vi "FourierSeries.vi"() -> ()   [LabVIEW 2020]
uses:
  <vilib>/Analysis/2dsp.llb/Real FFT.vi
  <vilib>/measure/NI_MABase.lvlib
  <vilib>/Analysis/NI_AALPro.lvlib
panel:
  out "Square Wave 2":dbl[](graph)
  out "FFT {X}":cdb[](array[numeric])
  out "Square Wave":waveform(dbl)(graph)
  in  "Frequency 2":dbl
  in  "Frequency":dbl
  in  "K":dbl
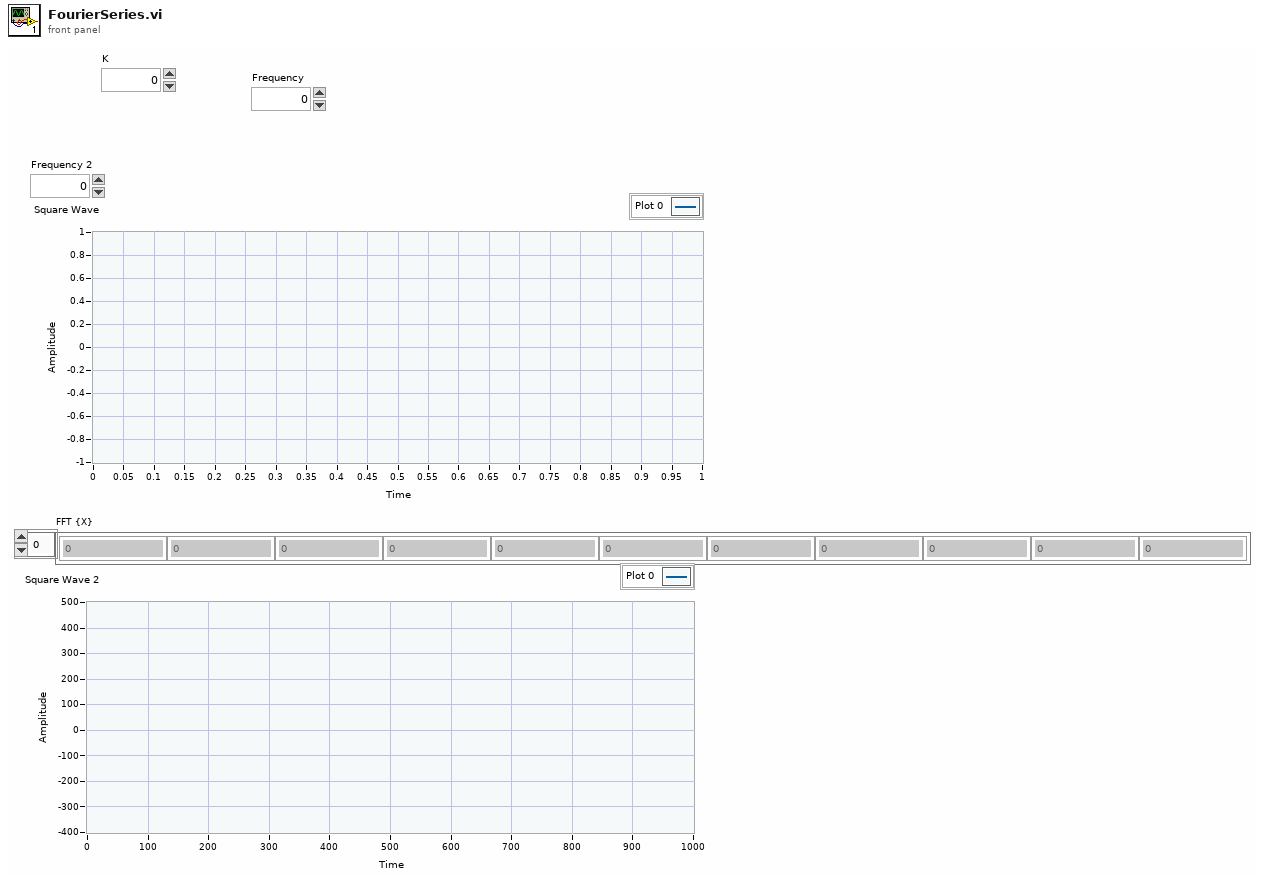
[diagram p1: front panel]
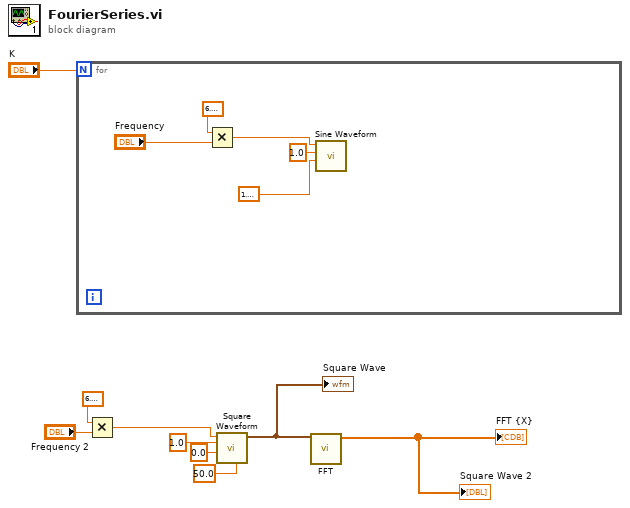
[diagram p0: block diagram]
diagram:
  n1 = for {
    N: "K" -> [_]
    n2 = Multiply(x=6.283185307179586, y="Frequency") -> (x*y=w10:dbl)
    n3 = call <vilib>:"Sine Waveform.vi"("phase"=1.5707963267948966, "amplitude"=1.0, "frequency"=w10) -> ()  [unwired: 7 in, 2 out]
  }
  n4 = Multiply(x=6.283185307179586, y="Frequency 2") -> (x*y=w4:dbl)
  n5 = call <vilib>:"Square Waveform.vi"("duty cycle (%)"=50.0, "phase"=0.0, "amplitude"=1.0, "frequency"=w4) -> ("signal out"=w2:waveform(dbl))  [unwired: 6 in, 1 out]
  "Square Wave" <- w2
  n6 = call-poly <vilib>:"FFT.vi"("X"=w2) -> ("FFT {X}"=→"FFT {X}" →"Square Wave 2":cdb[])  [unwired: 9 in, 1 out]
